vi "Read message.vi"(8 "error in (no error)":errorcluster, 9 "timeout in ms (10)":i32=10, 11 "Module queue ref":T3) -> (0 "error out":errorcluster, 3 "MSG to magnet":T1={"Command"=enum."Ignore", "Data"=variant(enum16{"Ramping", "Perzistant"} enum."Ramping")})   [LabVIEW 2022 SP3, in "Magnet module.lvlib"]
doc: "Reads message recived by magnet module. If timeout expire, result will be \"ignore\" command."
uses:
  Magnet module.lvlib
  Messenger service/Data types/Mailbox address.ctl
  ctl/MSG to magnet.ctl
  ctl/Magnet Orders.ctl
  Messenger service/MessengerLib.lvlib
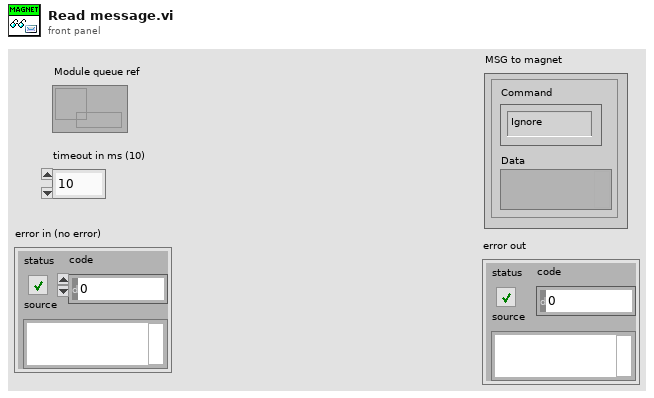
[diagram p1: front panel]
types:
  T1 = typedef "Magnet module.lvlib/MSG to magnet.ctl" = cluster{"Command":T2, "Data":variant}
  T2 = typedef "Magnet module.lvlib/Magnet Orders.ctl" = enum16{"Ignore", "Connect", "Update", "Switch mode", "Set field", "Stop ramping", "Equalize output", "Zero output", "Flip polarity", "Blackout", "Set timer", "Eval temperatures", "Disconnect"}
  T3 = typedef "MessengerLib.lvlib/Mailbox address.ctl" = refnum<queue>
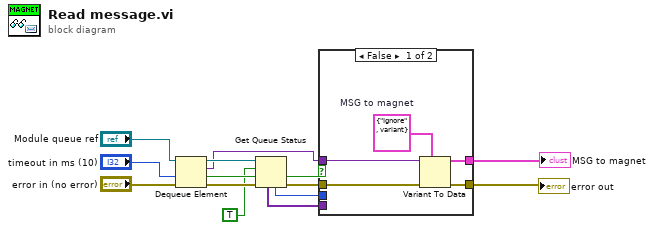
[diagram p0: block diagram]
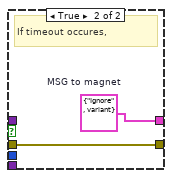
[diagram p2: hidden frame]
diagram:
  n1 = Dequeue Element(queue="Module queue ref", timeout in ms (-1)="timeout in ms (10)", error in (no error)="error in (no error)") -> (queue out=w8:T3, element=w2:variant, timed out?=w4:bool, error out=w5:errorcluster)
  n2 = Get Queue Status(queue=w8, return elements? (F)=TRUE, error in (no error)=w5) -> (error out=w3:errorcluster, # elements in queue=w6:i32, elements=w7:variant[])  [unwired: 5 out]
  n3 = case shown="False" w4 {
    tunnel: w2 -> [w18 _]
    tunnel: w3 -> [w17 w20]
    tunnel: [w16 w20] -> w10
    tunnel: [w15 w19] -> w9
    tunnel: w7 -> [_ _]
    tunnel: w6 -> [_ _]
    frame False {
      w14 = T1 {"Command"=enum."Ignore", "Data"=variant(enum16{"Ramping", "Perzistant"} enum."Ramping")}  # MSG to magnet
      n4 = Variant To Data(error in=w17, type=w14, Variant=w18) -> (data=w15:T1, error out=w16:errorcluster)
    }
    frame True {
      w19 = T1 {"Command"=enum."Ignore", "Data"=variant(enum16{"Ramping", "Perzistant"} enum."Ramping")}  # MSG to magnet
      # "If timeout occures,"
    }
  }
  "error out" <- w10
  "MSG to magnet" <- w9
